vi "Timer.vi"(7 "TimerState":enum16{"Reset", "Start", "GetTime", "Stop"}(ring), 8 "Error In":errorcluster, 11 "TargetTime(ms)":dbl format="%#_13g") -> (0 "Error Out":errorcluster, 3 "IsTimeElapsed":bool)   [LabVIEW 2019, in "Timer.lvlib"]
uses:
  Timer.lvlib
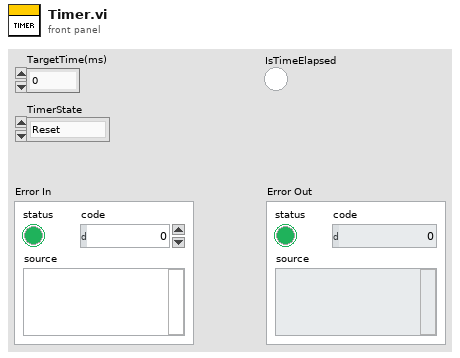
[diagram p1: front panel]
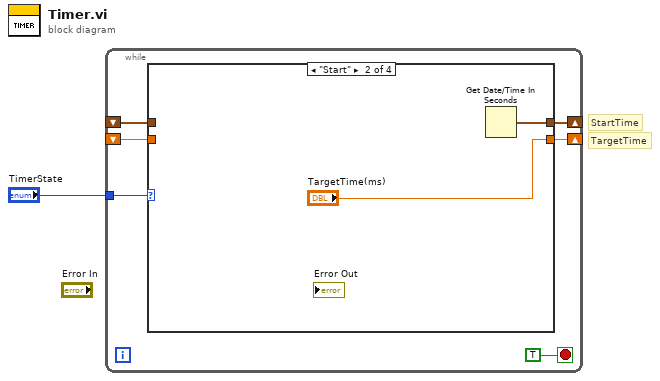
[diagram p0: block diagram]
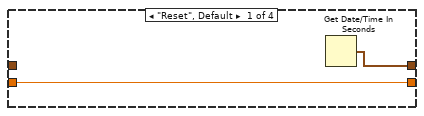
[diagram p2: hidden frame]
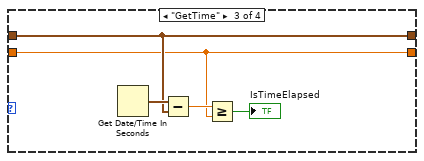
[diagram p3: hidden frame]
diagram:
  # "TargetTime"
  # "StartTime"
  n1 = while {
    tunnel: "TimerState" -> [w6]
    shift-right: [w5] -> _
    shift-left: _ -> [w4]
    shift-right: [w3] -> _
    shift-left: _ -> [w2]
    stop <- TRUE stop-if-true
    n2 = case shown="\"Start\"" w6 {
      tunnel: [w9 w11 w15 w18] -> w5
      tunnel: w4 -> [_ _ w15 w18]
      tunnel: [w8 "TargetTime(ms)" w13 w17] -> w3
      tunnel: w2 -> [w8 _ w13 w17]
      frame "Reset", Default {
        n3 = Get Date/Time In Seconds() -> (seconds since 1Jan1904=w9:timestamp)
      }
      frame "Start" {
        n4 = Get Date/Time In Seconds() -> (seconds since 1Jan1904=w11:timestamp)
      }
      frame "GetTime" {
        n5 = Get Date/Time In Seconds() -> (seconds since 1Jan1904=w16:timestamp)
        n6 = Subtract(x=w16, y=w15) -> (x-y=w14:dbl)
        n7 = Greater Or Equal?(x=w14, y=w13) -> (x >= y?=→"IsTimeElapsed":bool)
      }
      frame "Stop" {
      }
    }
  }
